vi "Motor controller.vi"() -> ()   [LabVIEW 2012]
uses:
  BotStatus.vi
panel:
  out "Transferable":bool
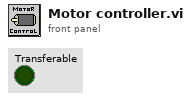
[diagram p1: front panel]
types:
  T1 = typedef "WPI_EncoderDevRef.ctl" = cluster{"DevStatus":errorcluster, "EncoderIndex":T2, "CounterIndex":T3, "DistancePerCount":dbl, "Decoding Type":T4}
  T2 = typedef "FPGA_EncoderIdx.ctl" = enum8{"Enc 0", "Enc 1", "Enc 2", "Enc 3", "Invalid"}
  T3 = typedef "FPGA_CounterCtrSystemIndex.ctl" = enum8{"Ctr 0", "Ctr 1", "Ctr 2", "Ctr 3", "Ctr 4", "Ctr 5", "Ctr 6", "Ctr 7", "Invalid"}
  T4 = typedef "WPI_EncoderType.ctl" = enum16{"1x", "2x", "4x"}
  T5 = typedef "WPI_MotorControlDeviceRef.ctl" = cluster{"DeviceStatus":errorcluster, "Type":enum16{"PWM", "CAN"}, "PWM":cluster{"Digital Module":T6, "PWM Channel":T7, "DeadBand":T8}, "CAN":cluster{"Device Number":u8, "Control Mode":T9, "Semaphore":T10, "Max Vout":dbl}, "Invert":bool, "TransformRef":T11, "InvTransformRef":T11}
  T6 = typedef "FPGA_TypedefDigitalModule.ctl" = enum16{"Digital Module 1", "Digital Module 2"}
  T7 = typedef "FPGA_DIOPWMChannel.ctl" = enum8{"PWM 1", "PWM 2", "PWM 3", "PWM 4", "PWM 5", "PWM 6", "PWM 7", "PWM 8", "PWM 9", "PWM 10", "Invalid"}
  T8 = typedef "WPI_PWMDeadband.ctl" = cluster{"Name":string, "maxPositivePwm":i32, "minPositivePwm":i32, "centerPwm":i32, "maxNegativePwm":i32, "minNegativePwm":i32, "angularRange":u16}
  T9 = typedef "WPI_CANJaguar_ControlMode.ctl" = enum8{"Percent VBus", "Current", "Speed", "Position", "Voltage"}
  T10 = typedef "Semaphore RefNum" = refnum<k1>
  T11 = typedef "WPI_PWMTransform_ConPane.ctl" = refnum<vi>
  T12 = typedef "WPI_ServoDeviceRef.ctl" = cluster{"DeviceStatus":errorcluster, "Digital Module":T6, "PWM Channel":T7, "DeadBand":T8}
  T13 = cluster{"Cannon Upper LS":bool, "Cannon Lower LS":bool}
  T14 = typedef "WPI_DigitalInputDevRef.ctl" = cluster{"DevStatus":errorcluster, "DIO Channel":T15, "Digital Module":T6}
  T15 = typedef "FPGA_DIOChannel.ctl" = enum8{"DIO 1", "DIO 2", "DIO 3", "DIO 4", "DIO 5", "DIO 6", "DIO 7", "DIO 8", "DIO 9", "DIO 10", "DIO 11", "DIO 12", "DIO 13", "DIO 14", "Invalid"}
  T16 = typedef "WPI_RelayDevRef.ctl" = cluster{"DevStatus":errorcluster, "Relay Channel":T17, "Digital Module":T6, "Relay Direction":T18}
  T17 = typedef "FPGA_DIORelayChannel.ctl" = enum8{"Relay 1", "Relay 2", "Relay 3", "Relay 4", "Relay 5", "Relay 6", "Relay 7", "Relay 8", "Invalid"}
  T18 = typedef "WPI_RelayDirection.ctl" = enum16{"Both directions", "Forward only", "Reverse only"}
  T19 = typedef "WPI_RelayValue.ctl" = enum16{"Off", "On", "Forward", "Reverse"}
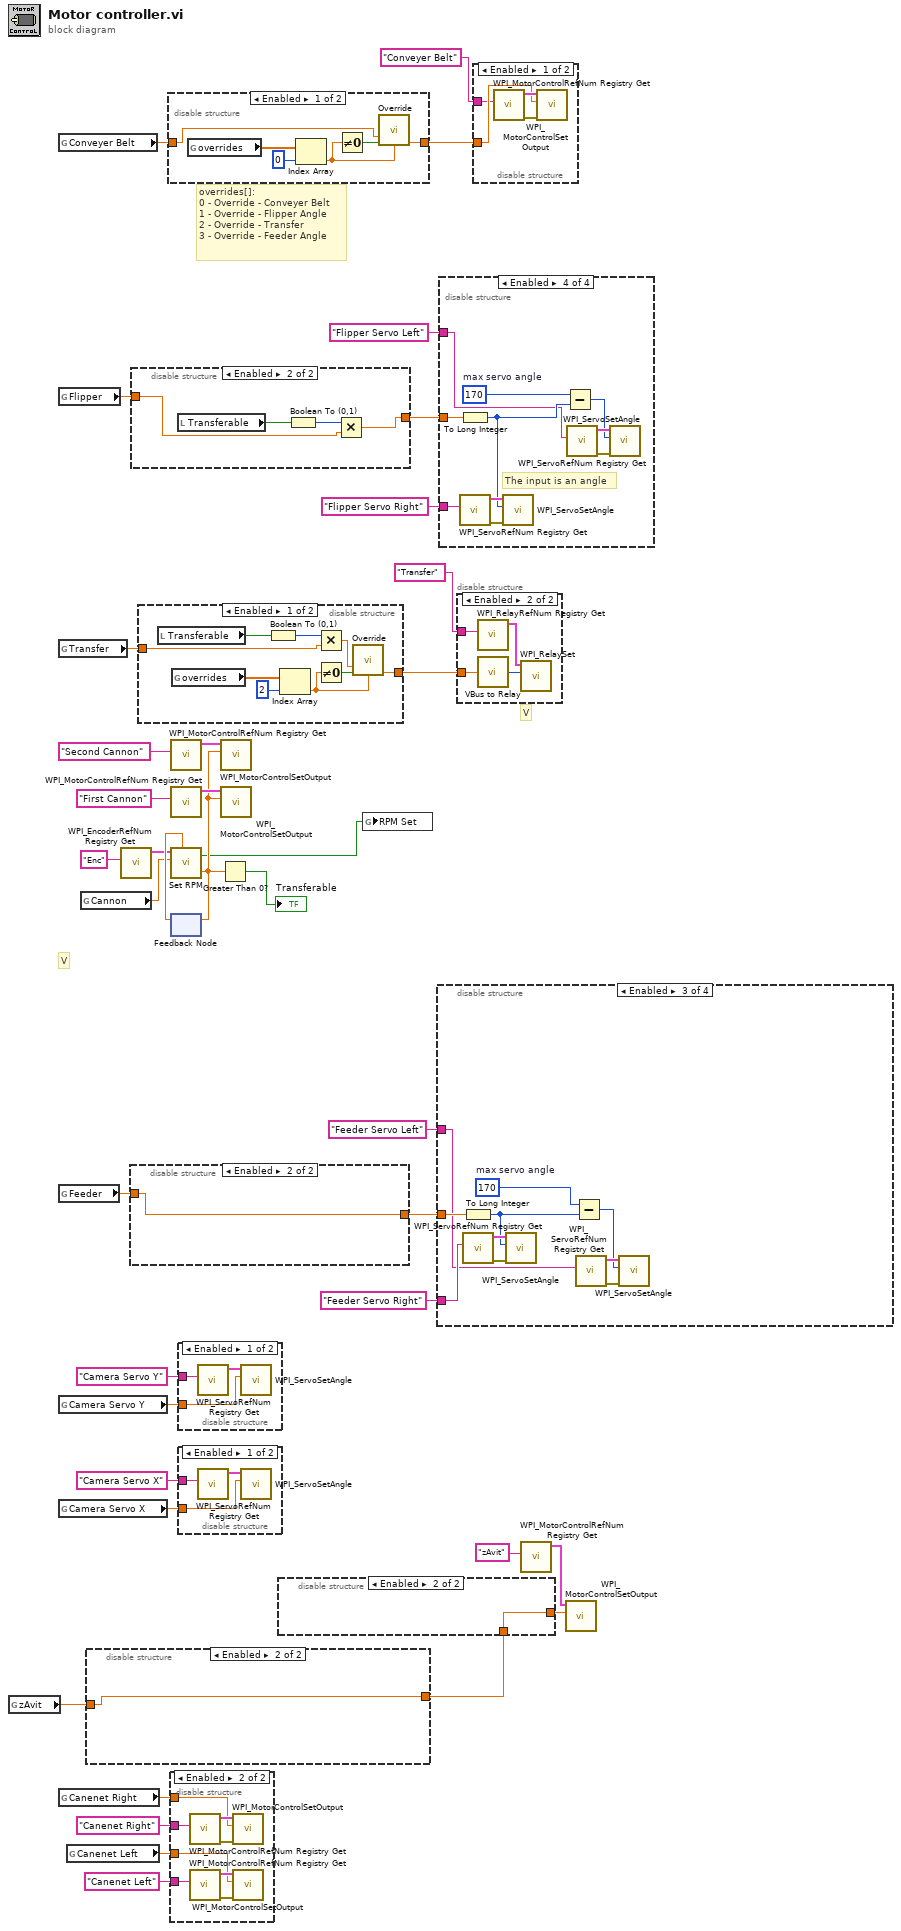
[diagram p0: block diagram]
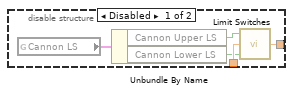
[diagram p2: hidden frame]
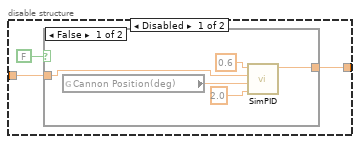
[diagram p3: hidden frame]
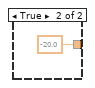
[diagram p4: hidden frame]
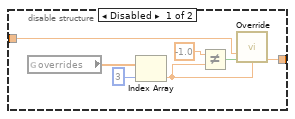
[diagram p7: hidden frame]
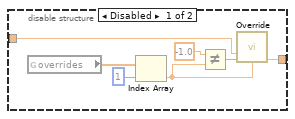
[diagram p9: hidden frame]
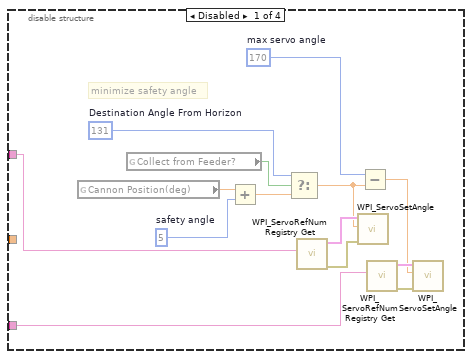
[diagram p12: hidden frame]
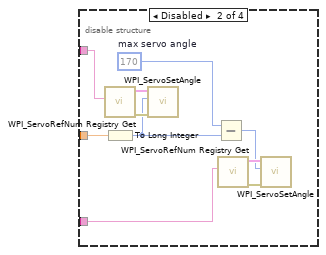
[diagram p13: hidden frame]
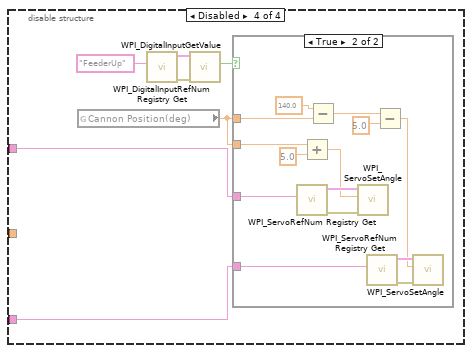
[diagram p14: hidden frame]
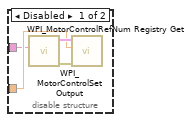
[diagram p16: hidden frame]
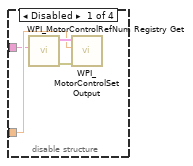
[diagram p17: hidden frame]
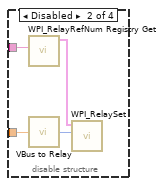
[diagram p18: hidden frame]
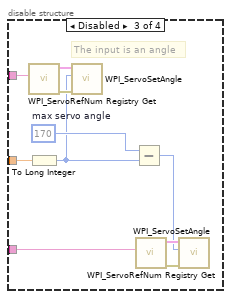
[diagram p19: hidden frame]
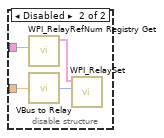
[diagram p20: hidden frame]
diagram:
  # "overrides[]:\n0 - Override - Conveyer Belt\n1 - Override - Flipper Angle \n2 - Override - Transfer\n3 - Override - Feeder Angle"
  # "V"
  # "V"
  n1 = global read "BotStatus.vi" "zAvit"() -> (w20:dbl)
  n2 = global read "BotStatus.vi" "Conveyer Belt"() -> (w14:dbl)
  n3 = global read "BotStatus.vi" "Flipper"() -> (w15:dbl)
  n4 = global read "BotStatus.vi" "Transfer"() -> (w16:dbl)
  n5 = global read "BotStatus.vi" "Feeder"() -> (w17:dbl)
  n6 = global read "BotStatus.vi" "Camera Servo Y"() -> (w18:dbl)
  n7 = global read "BotStatus.vi" "Camera Servo X"() -> (w19:dbl)
  n8 = global read "BotStatus.vi" "Canenet Right"() -> (w12:dbl)
  n9 = global read "BotStatus.vi" "Canenet Left"() -> (w13:dbl)
  n10 = global read "BotStatus.vi" "Cannon"() -> (w3:dbl)
  n11 = disable-structure shown="Enabled" {
    disable-tunnel: [w41 w48] -> w23
    disable-tunnel: w20 -> [w40 w48]
    frame Disabled {
      n12 = case shown="False" FALSE {
        tunnel: [w42 -20.0 ("zAvit")] -> w41
        tunnel: w40 -> [w46 _]
        frame False {
          n13 = global read "BotStatus.vi" "Cannon Position(deg)"() -> (w45:dbl)
          n14 = call "SimPID.vi"("Range"=2.0, "Position"=w45, "Set Point"=w46, "Gain"=0.6) -> ("result"=w42:dbl)  [unwired: 5 in, 1 out]
        }
        frame True {
        }
      }
    }
    frame Enabled {
    }
  }
  n15 = call <vilib>:"WPI_EncoderRefNum Registry Get.vi"("refnum name"="Enc") -> ("EncoderDevRef"=w5:T1)  [unwired: 9 in, 1 out]
  n16 = disable-structure shown="Enabled" {
    disable-tunnel: [w55 w56] -> w24
    disable-tunnel: w17 -> [w49 w56]
    frame Disabled {
      n17 = global read "BotStatus.vi" "overrides"() -> (w54:dbl[])
      n18 = Index Array(array=w54, index=3) -> (element=w50:dbl)
      n19 = Not Equal?(x=-1.0, y=w50) -> (x != y?=w51:bool)
      n20 = call "Override.vi"("Regualer"=w49, "Override"=w51, "Overriden"=w50) -> ("Output"=w55:dbl)  [unwired: 12 in]
    }
    frame Enabled {
    }
  }
  n21 = disable-structure shown="Enabled" {
    disable-tunnel: w15 -> [w63 w65]
    disable-tunnel: [w62 w64] -> w26
    frame Disabled {
      n22 = global read "BotStatus.vi" "overrides"() -> (w61:dbl[])
      n23 = Index Array(array=w61, index=1) -> (element=w57:dbl)
      n24 = Not Equal?(x=-1.0, y=w57) -> (x != y?=w58:bool)
      n25 = call "Override.vi"("Regualer"=w63, "Override"=w58, "Overriden"=w57) -> ("Output"=w62:dbl)  [unwired: 12 in]
    }
    frame Enabled {
      n26 = local read "Transferable"() -> (w66:bool)
      n27 = Boolean To (0,1)(Boolean=w66) -> (0, 1=w67:i16)
      n28 = Multiply(x=w67, y=w65) -> (x*y=w64:dbl)
    }
  }
  n29 = disable-structure shown="Enabled" {
    disable-tunnel: w16 -> [w71 w77]
    disable-tunnel: [w75 w77] -> w25
    frame Enabled {
      n30 = local read "Transferable"() -> (w70:bool)
      n31 = global read "BotStatus.vi" "overrides"() -> (w74:dbl[])
      n32 = Boolean To (0,1)(Boolean=w70) -> (0, 1=w69:i16)
      n33 = Index Array(array=w74, index=2) -> (element=w73:dbl)
      n34 = Multiply(x=w69, y=w71) -> (x*y=w68:dbl)
      n35 = Not Equal To 0?(x=w73) -> (x != 0?=w76:bool)
      n36 = call "Override.vi"("Regualer"=w68, "Override"=w76, "Overriden"=w73) -> ("Output"=w75:dbl)  [unwired: 12 in]
    }
    frame Disabled {
    }
  }
  n37 = disable-structure shown="Enabled" {
    disable-tunnel: [w83 w84] -> w27
    disable-tunnel: w14 -> [w82 w84]
    frame Enabled {
      n38 = global read "BotStatus.vi" "overrides"() -> (w81:dbl[])
      n39 = Index Array(array=w81, index=0) -> (element=w78:dbl)
      n40 = Not Equal To 0?(x=w78) -> (x != 0?=w79:bool)
      n41 = call "Override.vi"("Regualer"=w82, "Override"=w79, "Overriden"=w78) -> ("Output"=w83:dbl)  [unwired: 12 in]
    }
    frame Disabled {
    }
  }
  n42 = call <vilib>:"WPI_MotorControlRefNum Registry Get.vi"("refnum name"="Second Cannon") -> ("MotorControlDevRef"=w8:T5)  [unwired: 9 in, 1 out]
  n43 = call <vilib>:"WPI_MotorControlRefNum Registry Get.vi"("refnum name"="First Cannon") -> ("MotorControlDevRef"=w9:T5)  [unwired: 9 in, 1 out]
  n44 = feedback #1() -> (w6:dbl)  [unwired: 1 in]
  n45 = call "Set RPM.vi"("EncoderDevRef"=w5, "Set Point RPM"=w3, "Previous Vbus"=w6) -> ("READY!"=w1:bool, "Vbus Out"=w4:dbl)  [unwired: 2 in]
  n46 = feedback-in #1(w4) -> ()
  n47 = disable-structure shown="Enabled" {
    disable-tunnel: "Canenet Right" ("refnum name") -> [_ w88]
    disable-tunnel: "Canenet Left" ("refnum name") -> [_ w87]
    disable-tunnel: w12 -> [_ w86]
    disable-tunnel: w13 -> [_ w85]
    frame Disabled {
    }
    frame Enabled {
      n48 = call <vilib>:"WPI_MotorControlRefNum Registry Get.vi"("refnum name"=w88) -> ("error out"=w92:errorcluster, "MotorControlDevRef"=w91:T5)  [unwired: 9 in]
      n49 = call <vilib>:"WPI_MotorControlRefNum Registry Get.vi"("refnum name"=w87) -> ("error out"=w89:errorcluster, "MotorControlDevRef"=w90:T5)  [unwired: 9 in]
      n50 = call <vilib>:"WPI_MotorControlSetOutput.vi"("error in (no error)"=w92, "Output"=w86, "MotorControlDevRef"=w91) -> ()  [unwired: 6 in, 3 out]
      n51 = call <vilib>:"WPI_MotorControlSetOutput.vi"("error in (no error)"=w89, "Output"=w85, "MotorControlDevRef"=w90) -> ()  [unwired: 6 in, 3 out]
    }
  }
  n52 = disable-structure shown="Enabled" {
    disable-tunnel: "Camera Servo Y" ("refnum name") -> [w95 _]
    disable-tunnel: w18 -> [w93 _]
    frame Enabled {
      n53 = call <vilib>:"WPI_ServoRefNum Registry Get.vi"("refnum name"=w95) -> ("ServoDeviceRef"=w94:T12)  [unwired: 9 in, 1 out]
      n54 = call <vilib>:"WPI_ServoSetAngle.vi"("Angle"=w93, "ServoDeviceRef"=w94) -> ()  [unwired: 8 in, 2 out]
    }
    frame Disabled {
    }
  }
  n55 = disable-structure shown="Enabled" {
    disable-tunnel: "Camera Servo X" ("refnum name") -> [w98 _]
    disable-tunnel: w19 -> [w96 _]
    frame Enabled {
      n56 = call <vilib>:"WPI_ServoRefNum Registry Get.vi"("refnum name"=w98) -> ("ServoDeviceRef"=w97:T12)  [unwired: 9 in, 1 out]
      n57 = call <vilib>:"WPI_ServoSetAngle.vi"("Angle"=w96, "ServoDeviceRef"=w97) -> ()  [unwired: 8 in, 2 out]
    }
    frame Disabled {
    }
  }
  n58 = Greater Than 0?(x=w4) -> (x > 0?=→"Transferable":bool)
  n59 = call <vilib>:"WPI_MotorControlSetOutput.vi"("Output"=w4, "MotorControlDevRef"=w8) -> ()  [unwired: 7 in, 3 out]
  n60 = call <vilib>:"WPI_MotorControlSetOutput.vi"("Output"=w4, "MotorControlDevRef"=w9) -> ()  [unwired: 7 in, 3 out]
  n61 = disable-structure shown="Enabled" {
    disable-tunnel: w23 -> [w103 w104]
    disable-tunnel: [w102 w104] -> w22
    frame Disabled {
      n62 = global read "BotStatus.vi" "Cannon LS"() -> (w99:T13)
      n63 = Unbundle By Name(w99) -> ("Cannon Upper LS"=w101:bool, "Cannon Lower LS"=w100:bool)
      n64 = call "Limit Switches.vi"("Backward Limit Switch"=w100, "VBus in"=w103, "Forward Limit Switch"=w101) -> ("VBus out"=w102:dbl)
    }
    frame Enabled {
    }
  }
  n65 = global write "BotStatus.vi" "RPM Set"(w1) -> ()
  n66 = disable-structure shown="Enabled" {
    disable-tunnel: "Feeder Servo Left" ("refnum name") -> [w115 w120 w129 w141]
    disable-tunnel: "Feeder Servo Right" ("refnum name") -> [w112 w119 w130 w140]
    disable-tunnel: w24 -> [_ w122 w132 _]
    frame Disabled {
      w107 = 131  # Destination Angle From Horizon
      w111 = 170  # max servo angle
      w116 = 5  # safety angle
      # "minimize safety angle"
      n67 = global read "BotStatus.vi" "Cannon Position(deg)"() -> (w105:dbl)
      n68 = global read "BotStatus.vi" "Collect from Feeder?"() -> (w106:bool)
      n69 = Add(x=w105, y=w116) -> (x+y=w108:dbl)
      n70 = Select(t=w107, s=w106, f=w108) -> (s? t:f=w109:dbl)
      n71 = call <vilib>:"WPI_ServoRefNum Registry Get.vi"("refnum name"=w115) -> ("error out"=w117:errorcluster, "ServoDeviceRef"=w118:T12)  [unwired: 9 in]
      n72 = call <vilib>:"WPI_ServoSetAngle.vi"("error in (no error)"=w117, "Angle"=w109, "ServoDeviceRef"=w118) -> ()  [unwired: 7 in, 2 out]
      n73 = Subtract(x=w111, y=w109) -> (x-y=w110:dbl)
      n74 = call <vilib>:"WPI_ServoRefNum Registry Get.vi"("refnum name"=w112) -> ("error out"=w113:errorcluster, "ServoDeviceRef"=w114:T12)  [unwired: 9 in]
      n75 = call <vilib>:"WPI_ServoSetAngle.vi"("error in (no error)"=w113, "Angle"=w110, "ServoDeviceRef"=w114) -> ()  [unwired: 7 in, 2 out]
    }
    frame Disabled {
      w124 = 170  # max servo angle
      n76 = call <vilib>:"WPI_ServoRefNum Registry Get.vi"("refnum name"=w120) -> ("error out"=w127:errorcluster, "ServoDeviceRef"=w128:T12)  [unwired: 9 in]
      n77 = To Long Integer(number=w122) -> (32bit integer=w121:i32)
      n78 = call <vilib>:"WPI_ServoSetAngle.vi"("error in (no error)"=w127, "Angle"=w121, "ServoDeviceRef"=w128) -> ()  [unwired: 7 in, 2 out]
      n79 = Subtract(x=w124, y=w121) -> (x-y=w123:i32)
      n80 = call <vilib>:"WPI_ServoRefNum Registry Get.vi"("refnum name"=w119) -> ("error out"=w125:errorcluster, "ServoDeviceRef"=w126:T12)  [unwired: 9 in]
      n81 = call <vilib>:"WPI_ServoSetAngle.vi"("error in (no error)"=w125, "Angle"=w123, "ServoDeviceRef"=w126) -> ()  [unwired: 7 in, 2 out]
    }
    frame Enabled {
      w134 = 170  # max servo angle
      n82 = To Long Integer(number=w132) -> (32bit integer=w131:i32)
      n83 = call <vilib>:"WPI_ServoRefNum Registry Get.vi"("refnum name"=w130) -> ("error out"=w137:errorcluster, "ServoDeviceRef"=w138:T12)  [unwired: 9 in]
      n84 = call <vilib>:"WPI_ServoSetAngle.vi"("error in (no error)"=w137, "Angle"=w131, "ServoDeviceRef"=w138) -> ()  [unwired: 7 in, 2 out]
      n85 = Subtract(x=w134, y=w131) -> (x-y=w133:i32)
      n86 = call <vilib>:"WPI_ServoRefNum Registry Get.vi"("refnum name"=w129) -> ("error out"=w135:errorcluster, "ServoDeviceRef"=w136:T12)  [unwired: 9 in]
      n87 = call <vilib>:"WPI_ServoSetAngle.vi"("error in (no error)"=w135, "Angle"=w133, "ServoDeviceRef"=w136) -> ()  [unwired: 7 in, 2 out]
    }
    frame Disabled {
      n88 = global read "BotStatus.vi" "Cannon Position(deg)"() -> (w139:dbl)
      n89 = call <vilib>:"WPI_DigitalInputRefNum Registry Get.vi"("refnum name"="FeederUp") -> ("error out"=w143:errorcluster, "DigitalInputDevRef"=w142:T14)  [unwired: 9 in]
      n90 = call <vilib>:"WPI_DigitalInputGetValue.vi"("error in (no error)"=w143, "DigitalInputDevRef"=w142) -> ("Value"=w145:bool)  [unwired: 7 in, 2 out]
      n91 = case shown="True" w145 {
        tunnel: w141 -> [_ w157]
        tunnel: w139 -> [_ w156]
        tunnel: w140 -> [_ w148]
        tunnel: w139 -> [_ w147]
        frame False {
        }
        frame True {
          n92 = call <vilib>:"WPI_ServoRefNum Registry Get.vi"("refnum name"=w157) -> ("error out"=w158:errorcluster, "ServoDeviceRef"=w159:T12)  [unwired: 9 in]
          n93 = Add(x=w156, y=5.0) -> (x+y=w154:dbl)
          n94 = Subtract(x=140.0, y=w147) -> (x-y=w152:dbl)
          n95 = call <vilib>:"WPI_ServoSetAngle.vi"("error in (no error)"=w158, "Angle"=w154, "ServoDeviceRef"=w159) -> ()  [unwired: 7 in, 2 out]
          n96 = call <vilib>:"WPI_ServoRefNum Registry Get.vi"("refnum name"=w148) -> ("error out"=w149:errorcluster, "ServoDeviceRef"=w150:T12)  [unwired: 9 in]
          n97 = Subtract(x=w152, y=5.0) -> (x-y=w146:dbl)
          n98 = call <vilib>:"WPI_ServoSetAngle.vi"("error in (no error)"=w149, "Angle"=w146, "ServoDeviceRef"=w150) -> ()  [unwired: 7 in, 2 out]
        }
      }
    }
  }
  n99 = disable-structure shown="Enabled" {
    disable-tunnel: w26 -> [w161 w164 w174 w185]
    disable-tunnel: "Flipper Servo Left" ("refnum name") -> [w160 w166 w177 w179]
    disable-tunnel: "Flipper Servo Right" ("refnum name") -> [_ _ w168 w178]
    frame Disabled {
      n100 = call <vilib>:"WPI_MotorControlRefNum Registry Get.vi"("refnum name"=w160) -> ("error out"=w163:errorcluster, "MotorControlDevRef"=w162:T5)  [unwired: 9 in]
      n101 = call <vilib>:"WPI_MotorControlSetOutput.vi"("error in (no error)"=w163, "Output"=w161, "MotorControlDevRef"=w162) -> ()  [unwired: 6 in, 3 out]
    }
    frame Disabled {
      n102 = call <vilib>:"WPI_RelayRefNum Registry Get.vi"("refnum name"=w166) -> ("RelayDevRef"=w165:T16)  [unwired: 9 in, 1 out]
      n103 = call "VBus to Relay.vi"("Motor VBus"=w164) -> ("RelayValue"=w167:T19)  [unwired: 3 in]
      n104 = call <vilib>:"WPI_RelaySet.vi"("RelayValue"=w167, "RelayDevRef"=w165) -> ()  [unwired: 8 in, 2 out]
    }
    frame Disabled {
      w171 = 170  # max servo angle
      # "The input is an angle"
      n105 = call <vilib>:"WPI_ServoRefNum Registry Get.vi"("refnum name"=w177) -> ("error out"=w175:errorcluster, "ServoDeviceRef"=w176:T12)  [unwired: 9 in]
      n106 = To Long Integer(number=w174) -> (32bit integer=w170:i32)
      n107 = call <vilib>:"WPI_ServoSetAngle.vi"("error in (no error)"=w175, "Angle"=w170, "ServoDeviceRef"=w176) -> ()  [unwired: 7 in, 2 out]
      n108 = Subtract(x=w171, y=w170) -> (x-y=w169:i32)
      n109 = call <vilib>:"WPI_ServoRefNum Registry Get.vi"("refnum name"=w168) -> ("error out"=w173:errorcluster, "ServoDeviceRef"=w172:T12)  [unwired: 9 in]
      n110 = call <vilib>:"WPI_ServoSetAngle.vi"("error in (no error)"=w173, "Angle"=w169, "ServoDeviceRef"=w172) -> ()  [unwired: 7 in, 2 out]
    }
    frame Enabled {
      w182 = 170  # max servo angle
      # "The input is an angle"
      n111 = To Long Integer(number=w185) -> (32bit integer=w181:i32)
      n112 = call <vilib>:"WPI_ServoRefNum Registry Get.vi"("refnum name"=w178) -> ("error out"=w186:errorcluster, "ServoDeviceRef"=w187:T12)  [unwired: 9 in]
      n113 = call <vilib>:"WPI_ServoSetAngle.vi"("error in (no error)"=w186, "Angle"=w181, "ServoDeviceRef"=w187) -> ()  [unwired: 7 in, 2 out]
      n114 = Subtract(x=w182, y=w181) -> (x-y=w180:i32)
      n115 = call <vilib>:"WPI_ServoRefNum Registry Get.vi"("refnum name"=w179) -> ("error out"=w184:errorcluster, "ServoDeviceRef"=w183:T12)  [unwired: 9 in]
      n116 = call <vilib>:"WPI_ServoSetAngle.vi"("error in (no error)"=w184, "Angle"=w180, "ServoDeviceRef"=w183) -> ()  [unwired: 7 in, 2 out]
    }
  }
  n117 = disable-structure shown="Enabled" {
    disable-tunnel: w25 -> [w189 w192]
    disable-tunnel: "Transfer" ("refnum name") -> [w188 w194]
    frame Disabled {
      n118 = call <vilib>:"WPI_MotorControlRefNum Registry Get.vi"("refnum name"=w188) -> ("error out"=w191:errorcluster, "MotorControlDevRef"=w190:T5)  [unwired: 9 in]
      n119 = call <vilib>:"WPI_MotorControlSetOutput.vi"("error in (no error)"=w191, "Output"=w189, "MotorControlDevRef"=w190) -> ()  [unwired: 6 in, 3 out]
    }
    frame Enabled {
      n120 = call <vilib>:"WPI_RelayRefNum Registry Get.vi"("refnum name"=w194) -> ("RelayDevRef"=w193:T16)  [unwired: 9 in, 1 out]
      n121 = call "VBus to Relay.vi"("Motor VBus"=w192) -> ("RelayValue"=w195:T19)  [unwired: 3 in]
      n122 = call <vilib>:"WPI_RelaySet.vi"("RelayValue"=w195, "RelayDevRef"=w193) -> ()  [unwired: 8 in, 2 out]
    }
  }
  n123 = disable-structure shown="Enabled" {
    disable-tunnel: w27 -> [w197 w200]
    disable-tunnel: "Conveyer Belt" ("refnum name") -> [w196 w202]
    frame Enabled {
      n124 = call <vilib>:"WPI_MotorControlRefNum Registry Get.vi"("refnum name"=w196) -> ("error out"=w199:errorcluster, "MotorControlDevRef"=w198:T5)  [unwired: 9 in]
      n125 = call <vilib>:"WPI_MotorControlSetOutput.vi"("error in (no error)"=w199, "Output"=w197, "MotorControlDevRef"=w198) -> ()  [unwired: 6 in, 3 out]
    }
    frame Disabled {
      n126 = call <vilib>:"WPI_RelayRefNum Registry Get.vi"("refnum name"=w202) -> ("RelayDevRef"=w201:T16)  [unwired: 9 in, 1 out]
      n127 = call "VBus to Relay.vi"("Motor VBus"=w200) -> ("RelayValue"=w203:T19)  [unwired: 3 in]
      n128 = call <vilib>:"WPI_RelaySet.vi"("RelayValue"=w203, "RelayDevRef"=w201) -> ()  [unwired: 8 in, 2 out]
    }
  }
  n129 = call <vilib>:"WPI_MotorControlRefNum Registry Get.vi"("refnum name"="zAvit") -> ("MotorControlDevRef"=w30:T5)  [unwired: 9 in, 1 out]
  n130 = call <vilib>:"WPI_MotorControlSetOutput.vi"("Output"=w22, "MotorControlDevRef"=w30) -> ()  [unwired: 7 in, 3 out]
